vi "Convert_DMS_to_Decimal_Degrees.vi"(1 "Seconds":i16, 2 "Minutes":i16, 3 "Degrees":i16) -> (0 "Decimal Degrees":sgl)   [LabVIEW 2014]
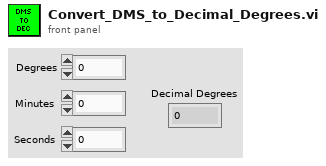
[diagram p1: front panel]
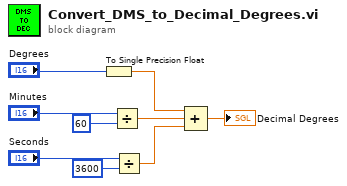
[diagram p0: block diagram]
diagram:
  n1 = To Single Precision Float(number="Degrees") -> (single precision float=w2:sgl)
  n2 = Divide(x="Minutes", y=i16 60) -> (x/y=w6:dbl)
  n3 = Divide(x="Seconds", y=i16 3600) -> (x/y=w3:dbl)
  n4 = Compound Arithmetic op=ADD(w2, w6, w3) -> (→"Decimal Degrees":dbl)
